vi "Parse Packet Data (EOF).vi"(8 "Error In":errorcluster, 10 "Recieved Bytes":u8[](array[numeric]), 11 "Packet Metadata In":T1 {"Server Status" format="%.0x"}) -> (0 "Error Out":errorcluster, 3 "Packet Metadata Out":T1 {"Server Status" format="%.0x"})   [LabVIEW 2014, in "hse-db.lvlib" / "MySQL (TCP).lvlib"]
uses:
  MySQL (TCP).lvlib
  Controls/OK Packet Metadata.ctl
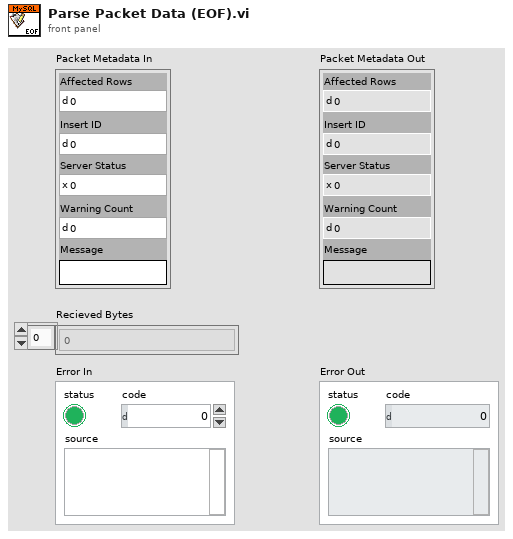
[diagram p1: front panel]
types:
  T1 = typedef "hse-db.lvlib/MySQL (TCP).lvlib/OK Packet Metadata.ctl" = cluster{"Affected Rows":u64, "Insert ID":u64, "Server Status":u16, "Warning Count":u16, "Message":string}
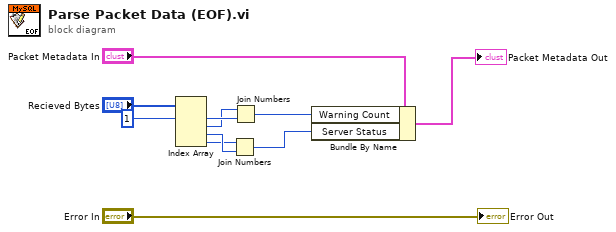
[diagram p0: block diagram]
diagram:
  n1 = Index Array(array="Recieved Bytes", index #1=1 ("Start Index")) -> (element #1=w9:u8, element #2=w8:u8, element #3=w6:u8, element #4=w5:u8)  [unwired: 3 in]
  n2 = Join Numbers(hi=w5, lo=w6) -> ((hi.lo)=w4:u16)
  n3 = Join Numbers(hi=w8, lo=w9) -> ((hi.lo)=w7:u16)
  n4 = Bundle By Name(cluster="Packet Metadata In", "Warning Count"=w7, "Server Status"=w4) -> (→"Packet Metadata Out":T1)
  "Error Out" <- "Error In"
